vi "Error Query (muliple).vi"(8 "error in (no error)":errorcluster, 11 "VISA resource name":refnum<visa-resource-name>) -> (0 "error out":errorcluster, 1 "Error Message":string, 2 "Error":i32[](array[numeric]), 3 "VISA resource name out":refnum<visa-resource-name>)   [LabVIEW 2015, in "Agilent 428X Series.lvlib"]
doc: "This VI reads the error queue from the instrument. It expects to see errors in SCPI format (#,\"error message\"). It continues to read from the error queue until it reads a 0, \"No error\". If the instrument does not support an error query, a warning is returned."
uses:
  <instrlib>/Agilent 428X Series/Agilent 428X Series.lvlib
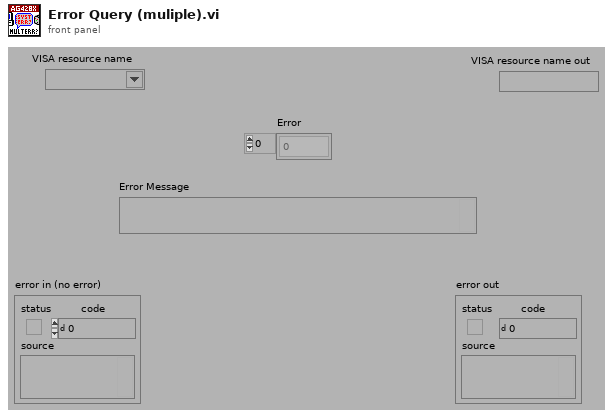
[diagram p1: front panel]
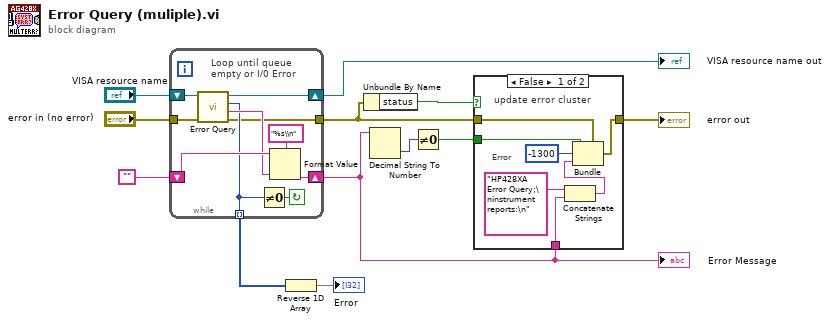
[diagram p0: block diagram]
diagram:
  n1 = while {
    tunnel: "error in (no error)" -> [w13]
    tunnel: [w16] -> w2 mode=indexing
    tunnel: [w14] -> w8
    shift-left: "VISA resource name" -> [w15]
    shift-right: [w22] -> w11
    shift-left: "" -> [w19]
    shift-right: [w21] -> w10
    stop <- w17 continue-if-true
    # "Loop until queue empty or I/0 Error"
    n2 = call <instrlib>:"Error Query.vi"("error in (no error)"=w13, "VISA resource name"=w15) -> ("error out"=w14:errorcluster, "Error Message"=w18:string, "Error"=w16:i32, "VISA resource name out"=w22:refnum<visa-resource-name>)  [unwired: 6 in]
    n3 = Not Equal To 0?(x=w16) -> (x != 0?=w17:bool)
    n4 = Format Value(string ("")=w19, format string="%s\\n", value (0)=w18) -> (output string=w21:string)
  }
  "Error Message" <- w10
  "VISA resource name out" <- w11
  n5 = Reverse 1D Array(array=w2) -> (reversed array=→"Error":i32[])
  n6 = Unbundle By Name(w8) -> ("status"=w5:bool)
  n7 = Decimal String To Number(string=w10) -> (number=w9:i32)  [unwired: 2 in, 1 out]
  n8 = Not Equal To 0?(x=w9) -> (x != 0?=w4:bool)
  n9 = case shown="False" w5 {
    tunnel: w8 -> [w28 w30]
    tunnel: [w27 w30] -> w6
    tunnel: w10 -> [w24 _]
    tunnel: w4 -> [w23 _]
    frame False {
      # "Error"
      # "update error cluster"
      n10 = Concatenate Strings("HP428XA Error Query;\ninstrument reports:\n", w24) -> (w26:string)
      n11 = Bundle(cluster=w28, "status"=w23, "code"=-1300, "source"=w26) -> (w27:errorcluster)
    }
    frame True {
      # "no instrument errors"
    }
  }
  "error out" <- w6
